vi "MAIN.vi"(8 "Error In":errorcluster, 9 "TLCamera reference out":refnum<k24>, 10 "TLCameraSDK reference out":refnum<k24>, 11 "MotorController out":refnum<class "MotorController.lvclass">) -> ()   [LabVIEW 2019]
doc: "Main control program for the C-Axis machine"
uses:
  MotorController.lvclass
  C:/Users/jleeman/git_repos/CAxis_Machine/C-Axis LabView Controller/Library_X64/Thorlabs.TSI.TLCameraInterfaces.dll
  Library_X64/Thorlabs.TSI.TLCameraInterfaces.dll
  main_enum_states_typedef.ctl
  enable_disable_enum_typedef.ctl
panel:
  in  "Shutdown":bool
  in  "Manual Jog":bool
  in  "Measure":bool
  in  "Scale Calibration":bool
  in  "Centroid Caliibration":bool
  in  "Align Polarizers":bool
  in  "Sample Calibration":bool
  in  "Set Camera":bool
  in  "Table Calibration":bool
  # "C-Axis Analyzer Control Panel"
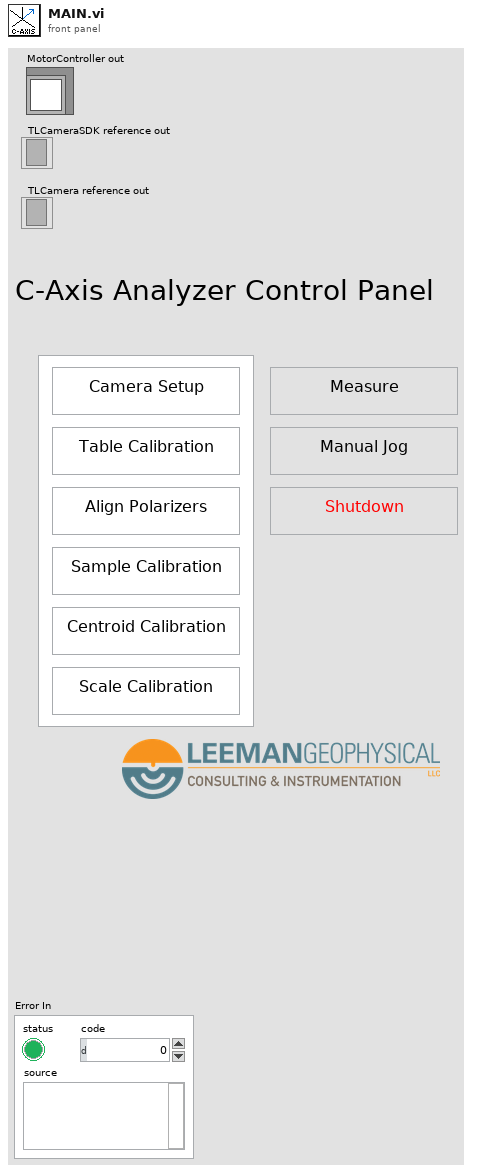
[diagram p1: front panel]
types:
  T1 = typedef "main_enum_states_typedef.ctl" = enum16{"Set Camera", "Initialize", "Sample Calibration", "Align Polarizers", "Centroid Calibration", "Scale Calibration", "Manual Jog", "Measure", "Table Calibration", "Wait", "Shutdown"}
  T2 = typedef "MotorController.lvclass/enable_disable_enum_typedef.ctl" = enum16{"Enable", "Disable"}
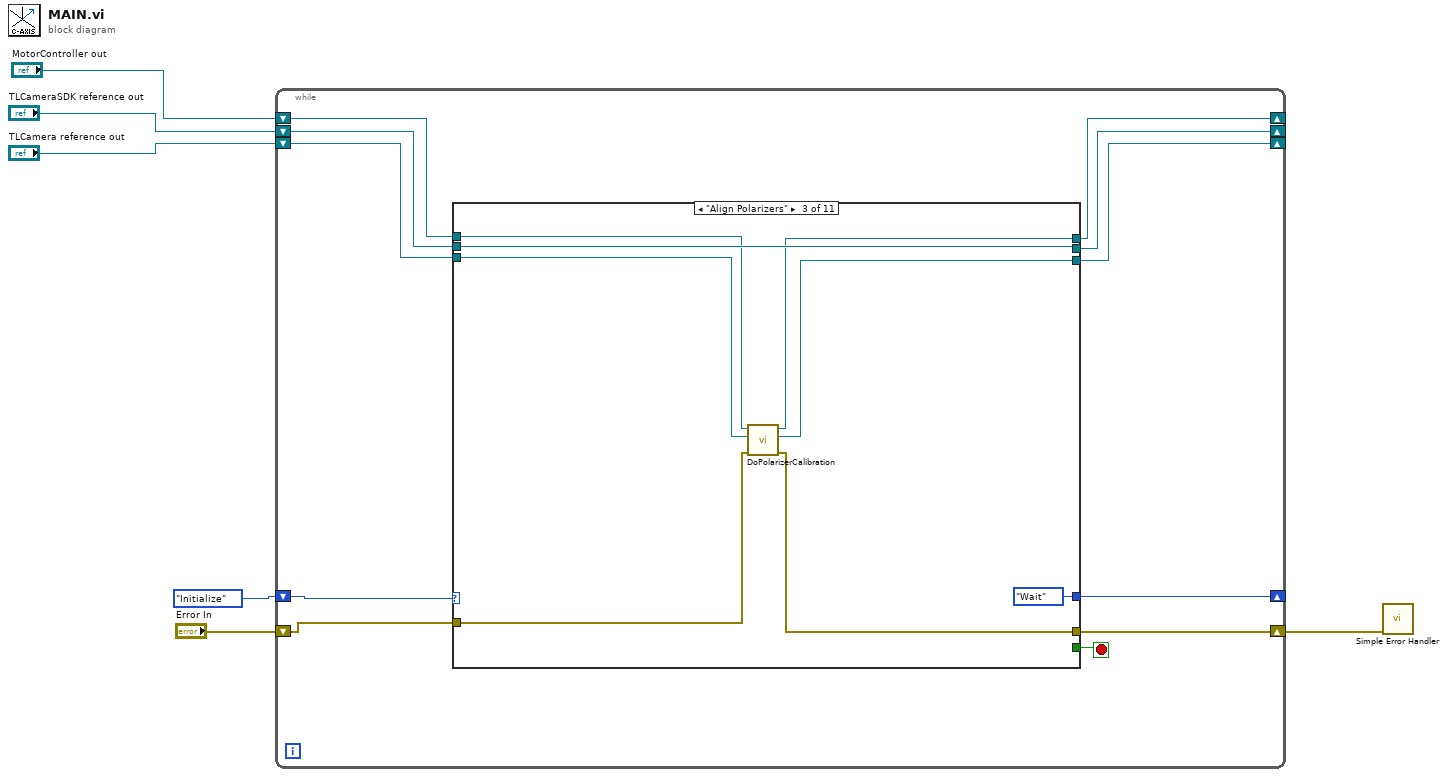
[diagram p0: block diagram]
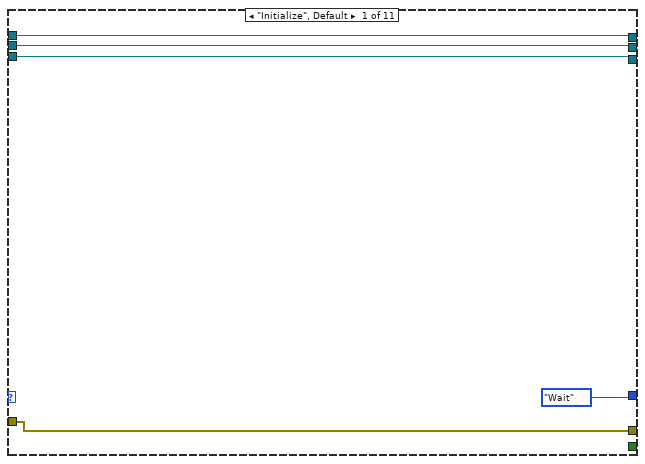
[diagram p2: hidden frame]
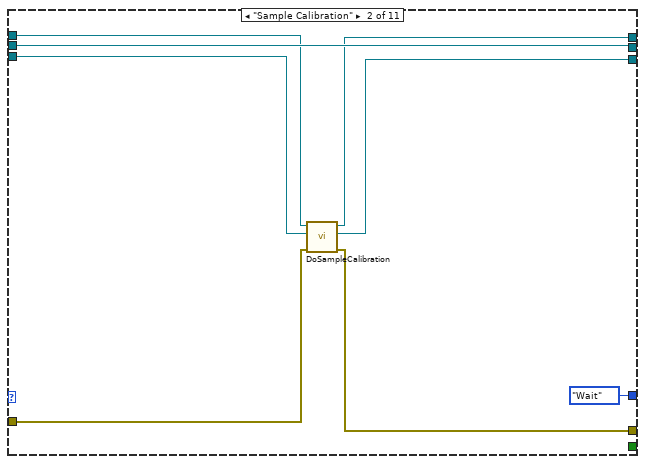
[diagram p3: hidden frame]
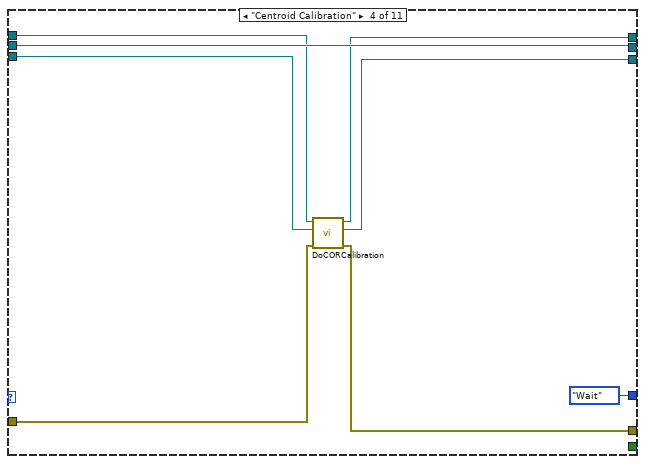
[diagram p4: hidden frame]
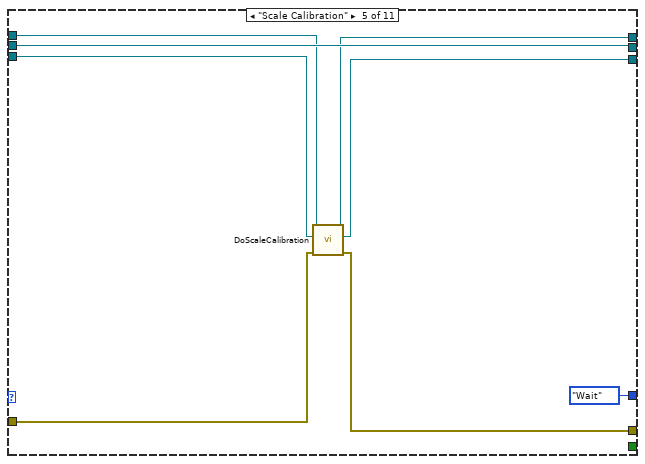
[diagram p5: hidden frame]
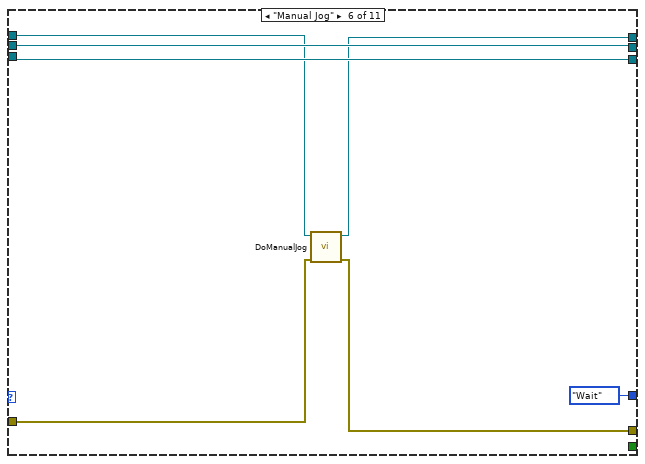
[diagram p6: hidden frame]
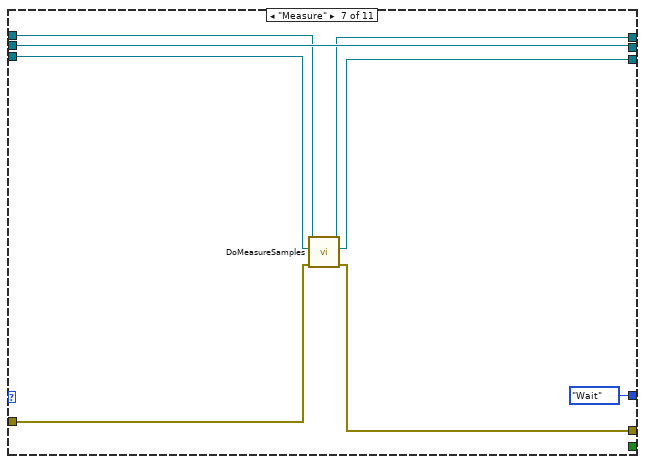
[diagram p7: hidden frame]
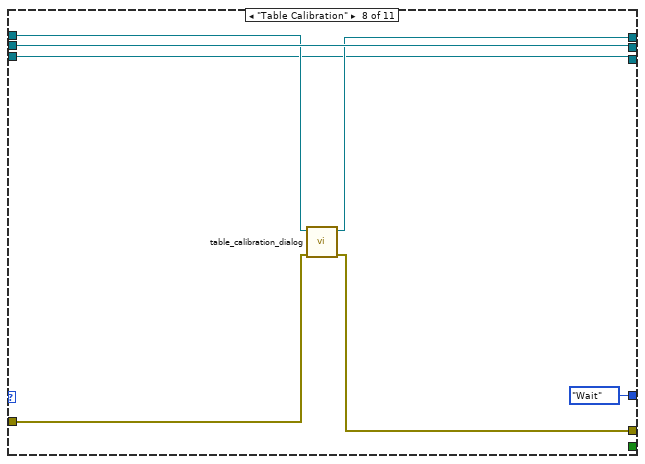
[diagram p8: hidden frame]
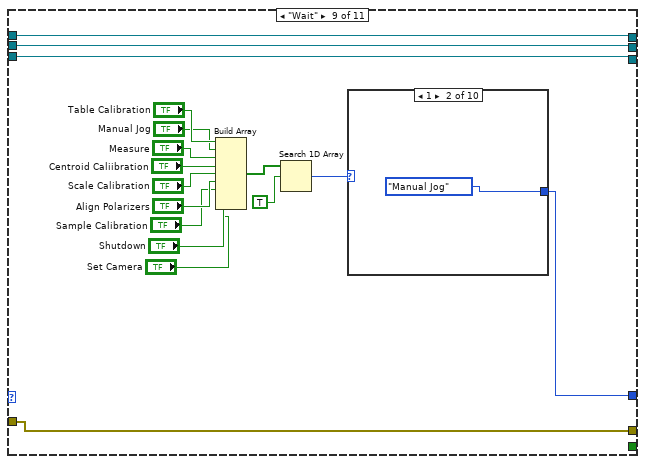
[diagram p9: hidden frame]
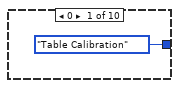
[diagram p10: hidden frame]
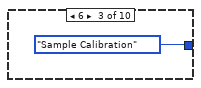
[diagram p11: hidden frame]
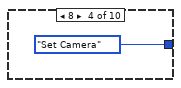
[diagram p12: hidden frame]
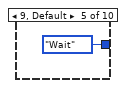
[diagram p13: hidden frame]
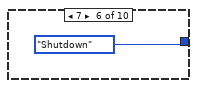
[diagram p14: hidden frame]
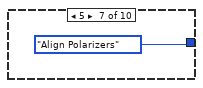
[diagram p15: hidden frame]
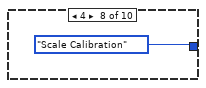
[diagram p16: hidden frame]
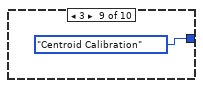
[diagram p17: hidden frame]
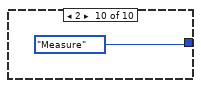
[diagram p18: hidden frame]
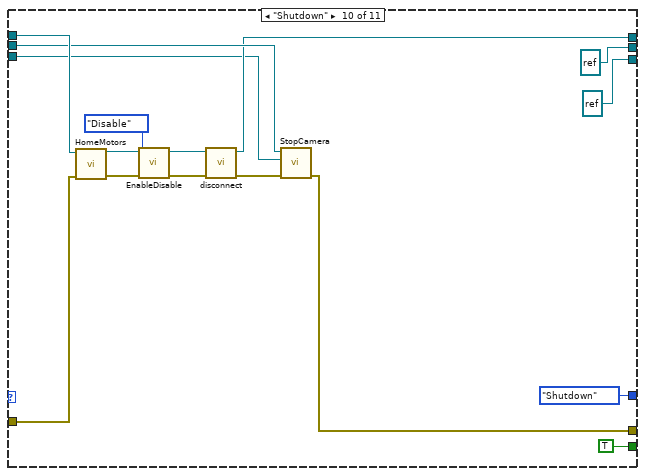
[diagram p19: hidden frame]
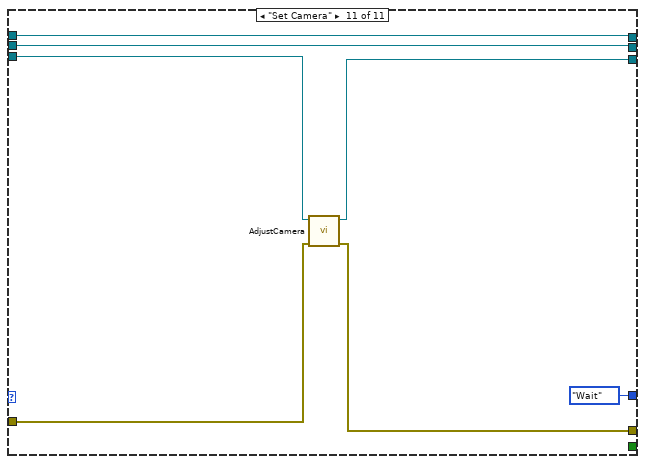
[diagram p20: hidden frame]
diagram:
  n1 = while {
    shift-right: [w16] -> _
    shift-left: main_enum_states_typedef."Initialize" -> [w17]
    shift-right: [w14] -> w4
    shift-left: "Error In" -> [w15]
    shift-right: [w13] -> _
    shift-left: "MotorController out" -> [w10]
    shift-right: [w12] -> _
    shift-left: "TLCameraSDK reference out" -> [w9]
    shift-right: [w11] -> _
    shift-left: "TLCamera reference out" -> [w8]
    stop <- w7 stop-if-true
    n2 = case shown="\"Align Polarizers\"" w17 {
      tunnel: [main_enum_states_typedef."Wait" main_enum_states_typedef."Wait" main_enum_states_typedef."Wait" main_enum_states_typedef."Wait" main_enum_states_typedef."Wait" main_enum_states_typedef."Wait" main_enum_states_typedef."Wait" main_enum_states_typedef."Wait" w78 main_enum_states_typedef."Shutdown" main_enum_states_typedef."Wait"] -> w16
      tunnel: w15 -> [w21 w25 w33 w42 w48 w56 w63 w71 w90 w107 w121]
      tunnel: [w21 w24 w32 w43 w47 w55 w62 w72 w90 w109 w122] -> w14
      tunnel: [w20 w28 w36 w44 w50 w57 w65 w74 w92 w111 w123] -> w13
      tunnel: [w19 w30 w38 w46 w54 w61 w69 w76 w93 refnum<k24> refnum ("TLCameraSDK reference out") w125] -> w12
      tunnel: [w18 w27 w35 w40 w51 w60 w66 w73 w91 refnum<k24> refnum ("TLCamera reference out") w124] -> w11
      tunnel: w10 -> [w20 w29 w37 w45 w49 w58 w64 w75 w92 w115 w123]
      tunnel: w9 -> [w19 w30 w38 w46 w54 w61 w69 w76 w93 w112 w125]
      tunnel: w8 -> [w18 w26 w34 w41 w52 w60 w67 w73 w91 w110 w126]
      tunnel: [_ _ _ _ _ _ _ _ _ TRUE _] -> w7
      frame "Initialize", Default {
      }
      frame "Sample Calibration" {
        n3 = call "DoSampleCalibration.vi"("Error In"=w25, "TLCamera reference in"=w26, "MotorController in"=w29) -> ("Error Out"=w24:errorcluster, "TLCamera reference out"=w27:refnum<k24>, "MotorController out"=w28:refnum<class "MotorController.lvclass">)  [unwired: 6 in]
      }
      frame "Align Polarizers" {
        n4 = call "DoPolarizerCalibration.vi"("Error In"=w33, "TLCamera reference in"=w34, "MotorController"=w37) -> ("Error Out"=w32:errorcluster, "TLCamera reference out"=w35:refnum<k24>, "MotorController Out"=w36:refnum<class "MotorController.lvclass">)  [unwired: 6 in]
      }
      frame "Centroid Calibration" {
        n5 = call "DoCORCalibration.vi"("Error In"=w42, "TLCamera reference in"=w41, "MotorController in"=w45) -> ("Error Out"=w43:errorcluster, "TLCamera reference out"=w40:refnum<k24>, "MotorController out"=w44:refnum<class "MotorController.lvclass">)  [unwired: 6 in]
      }
      frame "Scale Calibration" {
        n6 = call "DoScaleCalibration.vi"("Error In"=w48, "TLCamera reference in"=w52, "MotorController in"=w49) -> ("Error Out"=w47:errorcluster, "TLCamera reference out"=w51:refnum<k24>, "MotorController out"=w50:refnum<class "MotorController.lvclass">)  [unwired: 6 in]
      }
      frame "Manual Jog" {
        n7 = call "DoManualJog.vi"("Error In"=w56, "MotorController in"=w58) -> ("Error Out"=w55:errorcluster, "MotorController out"=w57:refnum<class "MotorController.lvclass">)  [unwired: 8 in]
      }
      frame "Measure" {
        n8 = call "DoMeasureSamples.vi"("Error In"=w63, "TLCamera reference in"=w67, "MotorController in"=w64) -> ("Error Out"=w62:errorcluster, "TLCamera reference out"=w66:refnum<k24>, "MotorController out"=w65:refnum<class "MotorController.lvclass">)  [unwired: 6 in]
      }
      frame "Table Calibration" {
        n9 = call "table_calibration_dialog.vi"("Error In"=w71, "MotorController"=w75) -> ("Error Out"=w72:errorcluster, "MotorController out"=w74:refnum<class "MotorController.lvclass">)  [unwired: 8 in]
      }
      frame "Wait" {
        n10 = Build Array("Table Calibration", "Manual Jog", "Measure", "Centroid Caliibration", "Scale Calibration", "Align Polarizers", "Sample Calibration", "Shutdown", "Set Camera") -> (w82:bool[])
        n11 = Search 1D Array(1D array=w82, element=TRUE) -> (index of element=w79:i32)  [unwired: 1 in]
        n12 = case shown="1" w79 {
          tunnel: [main_enum_states_typedef."Table Calibration" main_enum_states_typedef."Manual Jog" main_enum_states_typedef."Sample Calibration" main_enum_states_typedef."Set Camera" main_enum_states_typedef."Wait" main_enum_states_typedef."Shutdown" main_enum_states_typedef."Align Polarizers" main_enum_states_typedef."Scale Calibration" main_enum_states_typedef."Centroid Calibration" main_enum_states_typedef."Measure"] -> w78
          frame 0 {
          }
          frame 1 {
          }
          frame 6 {
          }
          frame 8 {
          }
          frame 9, Default {
          }
          frame 7 {
          }
          frame 5 {
          }
          frame 4 {
          }
          frame 3 {
          }
          frame 2 {
          }
        }
      }
      frame "Shutdown" {
        n13 = call "HomeMotors.vi"("error in (no error)"=w107, "MotorController in"=w115) -> ("error out"=w116:errorcluster, "MotorController out"=w119:refnum<class "MotorController.lvclass">)  [unwired: 8 in]
        n14 = call "EnableDisable.vi"("error in (no error)"=w116, "Action"=enable_disable_enum_typedef."Disable", "MotorController in"=w119) -> ("error out"=w117:errorcluster, "MotorController out"=w118:refnum<class "MotorController.lvclass">)  [unwired: 7 in]
        n15 = call "disconnect.vi"("error in (no error)"=w117, "MotorController in"=w118) -> ("error out"=w113:errorcluster, "MotorController out"=w111:refnum<class "MotorController.lvclass">)  [unwired: 8 in]
        n16 = call "StopCamera.vi"("Error In"=w113, "TLCamera reference"=w110, "TLCameraSDK reference"=w112) -> ("Error Out"=w109:errorcluster)  [unwired: 8 in]
      }
      frame "Set Camera" {
        n17 = call "AdjustCamera.vi"("Error In"=w121, "TLCamera reference in"=w126) -> ("Error Out"=w122:errorcluster, "TLCamera reference out"=w124:refnum<k24>)  [unwired: 7 in, 1 out]
      }
    }
  }
  n18 = call <vilib>:"Simple Error Handler.vi"("error in (no error)"=w4) -> ()  [unwired: 4 in, 5 out]
